vi "M14_Drive_Hardware_Globals.vi"() -> ()   [LabVIEW 2019]
panel:
  in  "Drive Right D Motor":string
  in  "Drive Right C Motor":string
  in  "Drive Left B Motor":string
  in  "Drive Left A Motor":string
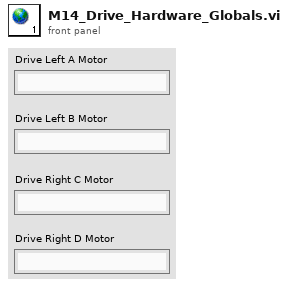
[diagram p1: front panel]
diagram:
